vi "SDCP Reset Connection.vi"(3 "error in (no error)":errorcluster, 4 "Frame byte":u8[](array[numeric]), 5 "COM Port":refnum<visa-resource-name>) -> (0 "error out":errorcluster, 1 "Active":bool, 2 "VISA out":refnum<visa-resource-name>)   [LabVIEW 2020]
uses:
  Typedefs/SDCP - Serial Port Control - Commands.ctl
  <vilib>/Instr/_visa.llb/VISA Flush IO Buffer Mask.ctl
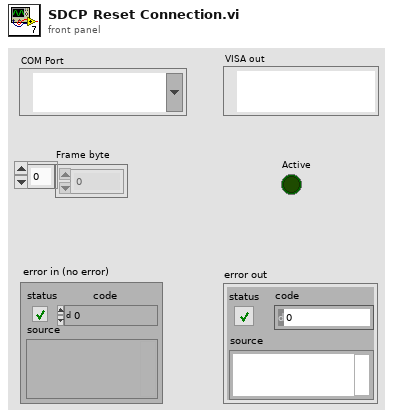
[diagram p1: front panel]
types:
  T1 = typedef "SDCP - Serial Port Control - Commands.ctl" = enum16{"Open", "Read", "Write", "Get instance", "Close"}
  T2 = typedef "VISA Flush IO Buffer Mask.ctl" = u16
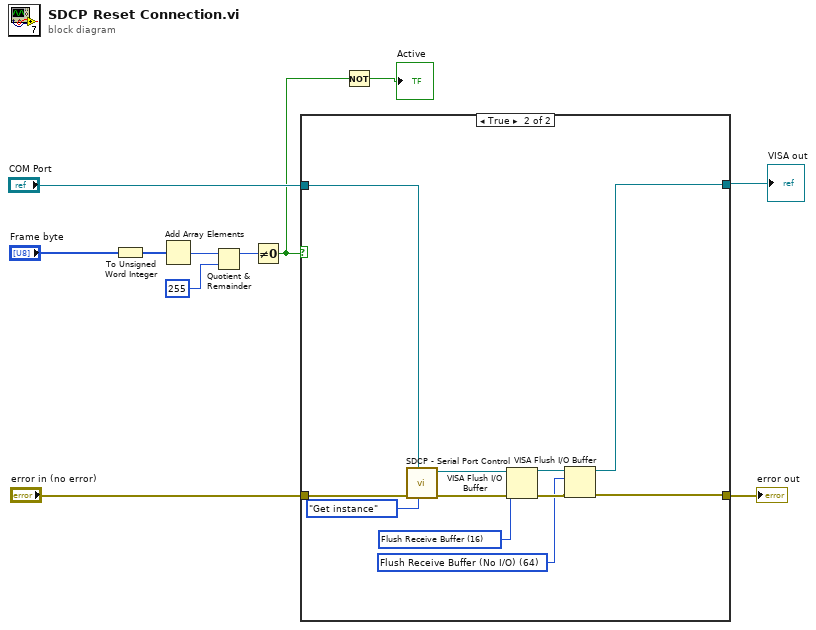
[diagram p0: block diagram]
diagram:
  n1 = To Unsigned Word Integer(number="Frame byte") -> ()  [unwired: 1 out]
  n2 = Add Array Elements(numeric array="Frame byte") -> (sum=w9:u8)
  n3 = Quotient & Remainder(x=w9, y=u8 255) -> (x-y*floor(x/y)=w7:u8)  [unwired: 1 out]
  n4 = Not Equal To 0?(x=w7) -> (x != 0?=w3:bool)
  n5 = case shown="True" w3 {
    tunnel: "COM Port" -> [w11 w21]
    tunnel: "error in (no error)" -> [w12 w23]
    tunnel: [w12 w13] -> w4
    tunnel: [w11 w14] -> w1
    frame False {
    }
    frame True {
      w17 = T2 64 items=["Flush Receive Buffer"=16, "Write Transmit Buffer to Device"=32, "Flush Receive Buffer (No I/O)"=64, "Flush Transmit Buffer"=128] ("Mask")
      w20 = T2 16 items=["Flush Receive Buffer"=16, "Write Transmit Buffer to Device"=32, "Flush Receive Buffer (No I/O)"=64, "Flush Transmit Buffer"=128] ("Mask")
      n6 = call "SDCP - Serial Port Control.vi"("Command"=SDCP_-_Serial_Port_Control_-_Commands."Get instance", "VISA resource name"=w21, "error in (no error)"=w23) -> ("error out"=w16:errorcluster, "VISA out"=w15:refnum<visa-resource-name>)  [unwired: 5 in, 2 out]
      n7 = VISA Flush I/O Buffer(VISA resource name=w15, mask (16)=w20, error in (no error)=w16) -> (VISA resource name out=w18:refnum<visa-resource-name>, error out=w19:errorcluster)
      n8 = VISA Flush I/O Buffer(VISA resource name=w18, mask (16)=w17, error in (no error)=w19) -> (VISA resource name out=w14:refnum<visa-resource-name>, error out=w13:errorcluster)
    }
  }
  "error out" <- w4
  "VISA out" <- w1
  n9 = Not(x=w3) -> (.not. x?=→"Active":bool)
